vi "Remove Header.vi"(8 "error in (no error)":errorcluster, 11 "HTTPHeaders_NET in":refnum<class "HttpHeaders_NET.lvclass">) -> (0 "error out":errorcluster, 3 "HTTPHeaders_NET out":refnum<class "HttpHeaders_NET.lvclass">)   [LabVIEW 2018, in "HttpClient_NET.lvlib" / "HttpHeaders_NET.lvclass"]
doc: "<b> </b> <b> </b>\nHttpClient_NET\nJustin Young - Viviota\nCopyright (c) 2021\nLicense: BSD"
uses:
  HttpHeaders_NET.lvclass
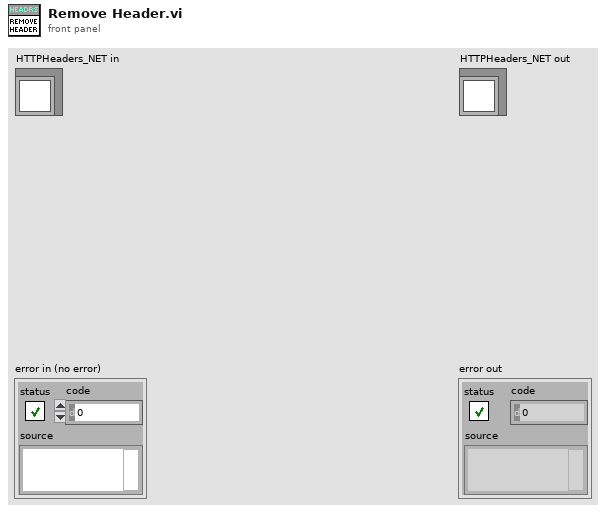
[diagram p1: front panel]
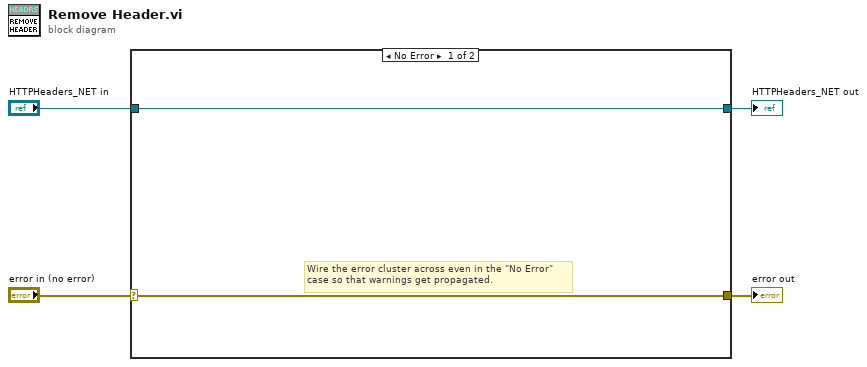
[diagram p0: block diagram]
diagram:
  n1 = case shown="No Error" "error in (no error)" {
    selector: "error in (no error)" -> [w5 w8]
    tunnel: [w5 w8] -> w3
    tunnel: [w6 w7] -> w1
    tunnel: "HTTPHeaders_NET in" -> [w6 w7]
    frame No Error {
      # "Wire the error cluster across even in the \"No Error\"\ncase so that warnings get propagated."
    }
    frame Error {
    }
  }
  "error out" <- w3
  "HTTPHeaders_NET out" <- w1
